vi "capex init.vi"(2 "GPIO registers":digitaldata={"transitions"=[], "data"=[[0, 0, 0, 0, 0, 0, 0, 0, 0, 0, 0, 0, 0, 0, 0, 0, 0, 0, 0, 0, 0, 0, 0, 0, 0, 0, 0, 0, 0, 0, 0, 0]]}) -> (0 "TC names default":string[](array[string]), 1 "DC defaults":dbl[](array[numeric]), 3 "AC defaults":dbl[](array[numeric]), 4 "Chiller defaults":dbl[](array[numeric]), 5 "AO names default":string[](array[string]), 6 "AI names default":string[](array[string]), 7 "Relay names default":string[](array[string]), 8 "AO defaults":dbl[](array[numeric]), 9 "Relay defaults":bool[](array[boolean]))   [LabVIEW 2013]
uses:
  <vilib>/Waveform/DTblOps.llb/DTbl Digital to Boolean Array.vi
  <resource>/objmgr/daqmx.rc
panel:
  in  "DC amps actual":dbl=60.0
  in  "DC volts actual":dbl=60.0
  in  "AC amps actual":dbl
  in  "AC volts actual":dbl
  in  "String 69":string="AI32"
  in  "String 68":string="AI31"
  in  "String 67":string="AI30"
  in  "String 66":string="AI29"
  in  "String 65":string="AI28"
  in  "String 64":string="AI27"
  in  "String 63":string="AI26"
  in  "String 62":string="AI25"
  in  "String 61":string="AI24"
  in  "String 60":string="AI23"
  in  "String 59":string="AI22"
  in  "String 58":string="AI21"
  in  "String 57":string="AI20"
  in  "String 56":string="AI19"
  in  "String 55":string="AI18"
  in  "String 54":string="AI17"
  in  "String 18":string="TC16"
  in  "String 17":string="TC15"
  out "hex integer string":string[](array[string])
  out "Array":tag[](array[tag])
  in  "Humidity process value":dbl
  in  "Temperature process value":dbl
  in  "Temperature setpoint":dbl
  in  "Humidity setpoint":dbl
  in  "String 53":string="Relay 4"
  in  "String 52":string="Relay 3"
  in  "String 51":string="Relay 2"
  in  "String 50":string="Relay 1"
  in  "String 49":string="AI16"
  in  "String 48":string="AI15"
  in  "String 47":string="AI14"
  in  "String 46":string="AI13"
  in  "String 45":string="AI12"
  in  "String 44":string="AI11"
  in  "String 43":string="AI10"
  in  "String 42":string="AI9"
  in  "String 41":string="AI8"
  in  "String 40":string="AI7"
  in  "String 39":string="AI6"
  in  "String 38":string="AI5"
  in  "String 37":string="AI4"
  in  "String 36":string="AI3"
  in  "String 35":string="AI2"
  in  "String 34":string="AI1"
  in  "Relay 4 default":bool
  in  "Relay 3 default":bool
  in  "Relay 2 default":bool
  in  "Relay 1 default":bool
  in  "Numeric 16":dbl
  in  "Numeric 15":dbl
  in  "Numeric 14":dbl
  in  "Numeric 13":dbl
  in  "Numeric 12":dbl
  in  "Numeric 11":dbl
  in  "Numeric 10":dbl
  in  "Numeric 9":dbl
  in  "Numeric 8":dbl
  in  "Numeric 7":dbl
  in  "Numeric 6":dbl
  in  "Numeric 5":dbl
  in  "Numeric 4":dbl
  in  "Numeric 3":dbl
  in  "Numeric 2":dbl
  in  "Numeric":dbl
  in  "String 33":string="AO16"
  in  "String 32":string="AO15"
  in  "String 31":string="AO14"
  in  "String 30":string="AO13"
  in  "String 29":string="AO12"
  in  "String 28":string="AO11"
  in  "String 27":string="AO10"
  in  "String 26":string="AO9"
  in  "String 25":string="AO8"
  in  "String 24":string="AO7"
  in  "String 23":string="AO6"
  in  "String 22":string="AO5"
  in  "String 21":string="AO4"
  in  "String 20":string="AO3"
  in  "String 19":string="AO2"
  in  "String 9":string="AO1"
  in  "Chiller pump default":dbl(ring) items=["Low", "Med", "High"]
  in  "Chiller temp default":dbl
  in  "DC OCP default":dbl
  in  "DC OVP default":dbl
  in  "DC amp default":dbl
  in  "DC volt default":dbl
  in  "AC frequency default":dbl=60.0
  in  "AC OCP default":dbl
  in  "AC OVP default":dbl
  in  "AC amp default":dbl
  in  "AC volt default":dbl
  in  "String 16":string="TC14"
  in  "String 15":string="TC13"
  in  "String 14":string="TC12"
  in  "String 13":string="TC11"
  in  "String 12":string="TC10"
  in  "String 11":string="TC9"
  in  "String 10":string="TC8"
  in  "String 8":string="TC7"
  in  "String 7":string="TC6"
  in  "String 6":string="TC5"
  in  "String 5":string="TC4"
  in  "String 4":string="TC3"
  in  "String 3":string="TC2"
  in  "String 2":string="TC1"
  # "Analog in"
  # "TC default names"
  # "Analog out"
  # "AC power starting values"
  # "DC power starting values"
  # "Chiller"
  # "Relays"
  # "Don't forget to set all items to default after editing!"
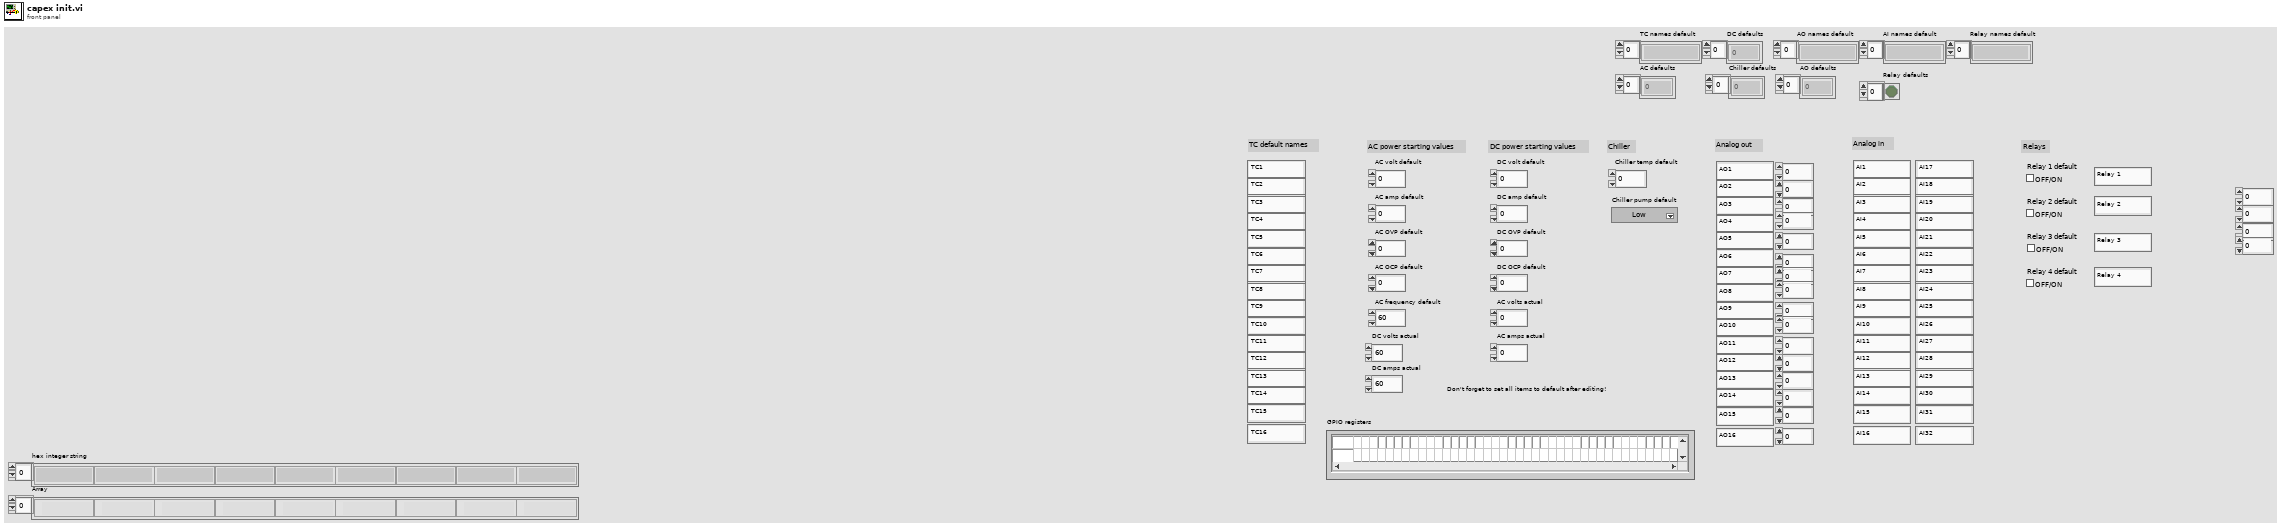
[diagram p1: front panel]
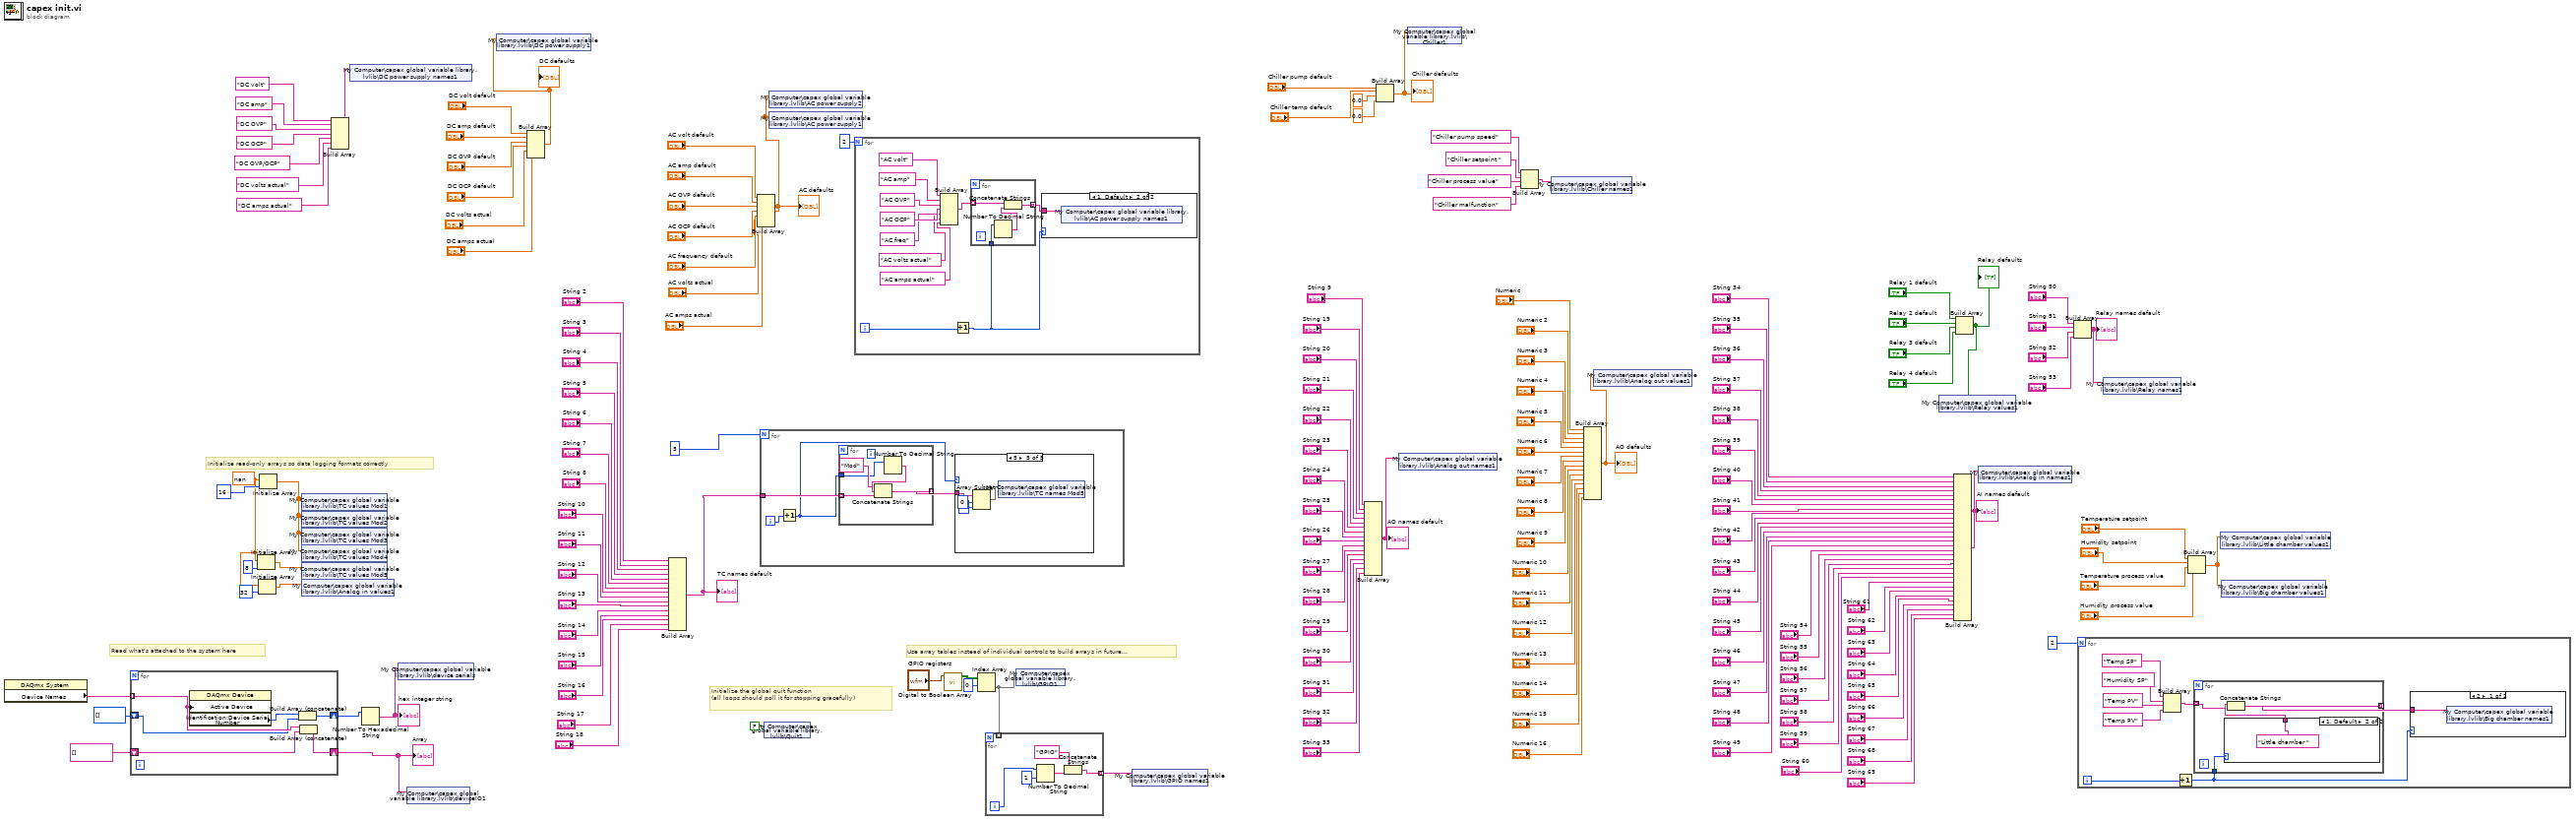
[diagram p0: block diagram]
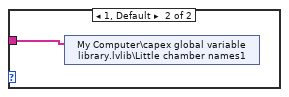
[diagram p2: hidden frame]
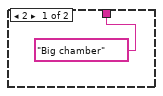
[diagram p3: hidden frame]
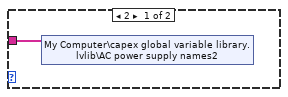
[diagram p4: hidden frame]
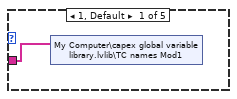
[diagram p5: hidden frame]
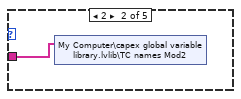
[diagram p6: hidden frame]
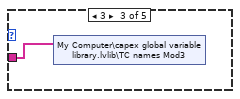
[diagram p7: hidden frame]
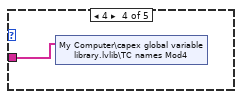
[diagram p8: hidden frame]
diagram:
  w27 = nan ("element")
  # "Initialize the global quit function\n(all loops should poll it for stopping gracefully)"
  # "Read what's attached to the system here"
  # "Initialize read-only arrays so data logging formats correctly"
  # "Use array tables instead of individual controls to build arrays in future..."
  n1 = property class="DAQmx System"() -> ("Device Names"=w36:tag[])  [unwired: 2 in, 2 out]
  n2 = for {
    tunnel: w36 -> [w159] mode=indexing
    shift-right: [w158] -> w32
    shift-left: tag[] [] -> [w160]
    shift-right: [w156] -> w34
    shift-left: u32[] [] -> [w155]
    n3 = property class="DAQmx Device"("Active Device"=w159) -> ("Identification:Device Serial Number"=w157:u32)  [unwired: 2 in, 2 out]
    n4 = Build Array (concatenate)(w157, w155) -> (w156:u32[])
    n5 = Build Array (concatenate)(w159, w160) -> (w158:tag[])
  }
  "Array" <- w32
  n6 = Initialize Array(w27, 8 ("dimension size")) -> (w29:dbl[])
  n7 = Initialize Array(w27, 32 ("dimension size")) -> (w28:dbl[])
  n8 = Initialize Array(w27, 16 ("dimension size")) -> (w37:dbl[])
  n9 = shared-variable "My Computer\\capex global variable library.lvlib\\TC values Mod1"(w37) -> ()  [unwired: 1 in, 1 out]
  n10 = shared-variable "My Computer\\capex global variable library.lvlib\\TC values Mod2"(w37) -> ()  [unwired: 1 in, 1 out]
  n11 = shared-variable "My Computer\\capex global variable library.lvlib\\TC values Mod3"(w37) -> ()  [unwired: 1 in, 1 out]
  n12 = shared-variable "My Computer\\capex global variable library.lvlib\\TC values Mod4"(w37) -> ()  [unwired: 1 in, 1 out]
  n13 = shared-variable "My Computer\\capex global variable library.lvlib\\TC values Mod5"(w29) -> ()  [unwired: 1 in, 1 out]
  n14 = shared-variable "My Computer\\capex global variable library.lvlib\\Analog in values1"(w28) -> ()  [unwired: 1 in, 1 out]
  n15 = Build Array("DC volt", "DC amp", "DC OVP", "DC OCP", "DC OVP/OCP", "DC volts actual", "DC amps actual") -> (w49:string[])
  n16 = shared-variable "My Computer\\capex global variable library.lvlib\\DC power supply names1"(w49) -> ()  [unwired: 1 in, 1 out]
  n17 = Number To Hexadecimal String(2:w34) -> (0:w31:string[])  [unwired: 1 in]
  "hex integer string" <- w31
  n18 = shared-variable "My Computer\\capex global variable library.lvlib\\device serials"(w31) -> ()  [unwired: 1 in, 1 out]
  n19 = shared-variable "My Computer\\capex global variable library.lvlib\\deviceIO1"(w32) -> ()  [unwired: 1 in, 1 out]
  n20 = Build Array("DC volt default", "DC amp default", "DC OVP default", "DC OCP default", "DC volts actual", "DC amps actual") -> (w70:dbl[])
  "DC defaults" <- w70
  n21 = shared-variable "My Computer\\capex global variable library.lvlib\\DC power supply1"(w70) -> ()  [unwired: 1 in, 1 out]
  n22 = Build Array("String 2", "String 3", "String 4", "String 5", "String 6", "String 7", "String 8", "String 10", "String 11", "String 12", "String 13", "String 14", "String 15", "String 16", "String 17", "String 18") -> (w73:string[])
  "TC names default" <- w73
  n23 = Build Array("AC volt default", "AC amp default", "AC OVP default", "AC OCP default", "AC frequency default", "AC volts actual", "AC amps actual") -> (w71:dbl[])
  "AC defaults" <- w71
  n24 = for {
    N: 5 -> [_]
    tunnel: w73 -> [w164]
    i -> [w162]
    n25 = Increment(x=w162) -> (x+1=w161:i32)
    n26 = for {
      tunnel: w164 -> [w177] mode=indexing
      tunnel: w161 -> [w174]
      tunnel: [w173] -> w163 mode=indexing
      n27 = Number To Decimal String(number=w174) -> (decimal integer string=w176:string)  [unwired: 1 in]
      n28 = Concatenate Strings("Mod" ("string"), w176, w177) -> (w173:string)
    }
    n29 = case shown="5" w161 {
      tunnel: w163 -> [w165 w166 w167 w168 w172]
      frame 1, Default {
        n30 = shared-variable "My Computer\\capex global variable library.lvlib\\TC names Mod1"(w165) -> ()  [unwired: 1 in, 1 out]
      }
      frame 2 {
        n31 = shared-variable "My Computer\\capex global variable library.lvlib\\TC names Mod2"(w166) -> ()  [unwired: 1 in, 1 out]
      }
      frame 3 {
        n32 = shared-variable "My Computer\\capex global variable library.lvlib\\TC names Mod3"(w167) -> ()  [unwired: 1 in, 1 out]
      }
      frame 4 {
        n33 = shared-variable "My Computer\\capex global variable library.lvlib\\TC names Mod4"(w168) -> ()  [unwired: 1 in, 1 out]
      }
      frame 5 {
        n34 = Array Subset(array=w172, index=0, length=8) -> (w169:string[])
        n35 = shared-variable "My Computer\\capex global variable library.lvlib\\TC names Mod5"(w169) -> ()  [unwired: 1 in, 1 out]
      }
    }
  }
  n36 = shared-variable "My Computer\\capex global variable library.lvlib\\Quit1"(FALSE ("Quit1")) -> ()  [unwired: 1 in, 1 out]
  n37 = shared-variable "My Computer\\capex global variable library.lvlib\\AC power supply2"(w71) -> ()  [unwired: 1 in, 1 out]
  n38 = shared-variable "My Computer\\capex global variable library.lvlib\\AC power supply1"(w71) -> ()  [unwired: 1 in, 1 out]
  n39 = for {
    N: 2 -> [_]
    i -> [w179]
    n40 = Build Array("AC volt", "AC amp", "AC OVP", "AC OCP", "AC freq", "AC volts actual", "AC amps actual") -> (w182:string[])
    n41 = Increment(x=w179) -> (x+1=w180:i32)
    n42 = for {
      tunnel: w182 -> [w194] mode=indexing
      tunnel: [w192] -> w181 mode=indexing
      tunnel: w180 -> [w191]
      n43 = Number To Decimal String(number=w191) -> (decimal integer string=w193:string)  [unwired: 1 in]
      n44 = Concatenate Strings(w194, w193) -> (w192:string)
    }
    n45 = case shown="1, Default" w180 {
      tunnel: w181 -> [w189 w190]
      frame 2 {
        n46 = shared-variable "My Computer\\capex global variable library.lvlib\\AC power supply names2"(w189) -> ()  [unwired: 1 in, 1 out]
      }
      frame 1, Default {
        n47 = shared-variable "My Computer\\capex global variable library.lvlib\\AC power supply names1"(w190) -> ()  [unwired: 1 in, 1 out]
      }
    }
  }
  n48 = call-poly <vilib>:"Digital to Boolean Array.vi"("digital data"="GPIO registers") -> ("boolean array"=w62:bool[][])  [unwired: 9 in, 1 out]
  n49 = Index Array(array=w62, index (row)=0) -> (element=w43:bool[])  [unwired: 1 in]
  n50 = for {
    tunnel: w43 -> [_] mode=indexing
    tunnel: [w195] -> w42 mode=indexing
    i -> [w196]
    n51 = Number To Decimal String(number=w196, width (-)=i16 1) -> (decimal integer string=w198:string)
    n52 = Concatenate Strings("GPIO" ("string"), w198) -> (w195:string)
  }
  n53 = shared-variable "My Computer\\capex global variable library.lvlib\\GPIO1"(w43) -> ()  [unwired: 1 in, 1 out]
  n54 = shared-variable "My Computer\\capex global variable library.lvlib\\GPIO names1"(w42) -> ()  [unwired: 1 in, 1 out]
  n55 = Build Array("String 9", "String 19", "String 20", "String 21", "String 22", "String 23", "String 24", "String 25", "String 26", "String 27", "String 28", "String 29", "String 30", "String 31", "String 32", "String 33") -> (w68:string[])
  "AO names default" <- w68
  n56 = Build Array("Chiller pump default", "Chiller temp default", 0.0 ("element"), 0.0 ("element")) -> (w69:dbl[])
  "Chiller defaults" <- w69
  n57 = shared-variable "My Computer\\capex global variable library.lvlib\\Analog out names1"(w68) -> ()  [unwired: 1 in, 1 out]
  n58 = shared-variable "My Computer\\capex global variable library.lvlib\\Chiller1"(w69) -> ()  [unwired: 1 in, 1 out]
  n59 = Build Array("Chiller pump speed", "Chiller setpoint ", "Chiller process value", "Chiller malfunction") -> (w44:string[])
  n60 = shared-variable "My Computer\\capex global variable library.lvlib\\Chiller names1"(w44) -> ()  [unwired: 1 in, 1 out]
  n61 = Build Array("Numeric", "Numeric 2", "Numeric 3", "Numeric 4", "Numeric 5", "Numeric 6", "Numeric 7", "Numeric 8", "Numeric 9", "Numeric 10", "Numeric 11", "Numeric 12", "Numeric 13", "Numeric 14", "Numeric 15", "Numeric 16") -> (w67:dbl[])
  "AO defaults" <- w67
  n62 = shared-variable "My Computer\\capex global variable library.lvlib\\Analog out values1"(w67) -> ()  [unwired: 1 in, 1 out]
  n63 = Build Array("String 34", "String 35", "String 36", "String 37", "String 38", "String 39", "String 40", "String 41", "String 42", "String 43", "String 44", "String 45", "String 46", "String 47", "String 48", "String 49", "String 54", "String 55", "String 56", "String 57", "String 58", "String 59", "String 60", "String 61", "String 62", "String 63", "String 64", "String 65", "String 66", "String 67", "String 68", "String 69") -> (w66:string[])
  "AI names default" <- w66
  n64 = Build Array("Relay 1 default", "Relay 2 default", "Relay 3 default", "Relay 4 default") -> (w65:bool[])
  "Relay defaults" <- w65
  n65 = shared-variable "My Computer\\capex global variable library.lvlib\\Relay values1"(w65) -> ()  [unwired: 1 in, 1 out]
  n66 = shared-variable "My Computer\\capex global variable library.lvlib\\Analog in names1"(w66) -> ()  [unwired: 1 in, 1 out]
  n67 = Build Array("String 50", "String 51", "String 52", "String 53") -> (w64:string[])
  "Relay names default" <- w64
  n68 = for {
    N: 2 -> [_]
    i -> [w201]
    n69 = Build Array("Temp SP", "Humidity SP", "Temp PV", "Temp PV") -> (w203:string[])
    n70 = Increment(x=w201) -> (x+1=w200:i32)
    n71 = for {
      tunnel: w203 -> [w210] mode=indexing
      tunnel: [w213] -> w202 mode=indexing
      tunnel: w200 -> [w212]
      n72 = case shown="1, Default" w212 {
        tunnel: ["Big chamber" "Little chamber "] -> w211
        frame 2 {
        }
        frame 1, Default {
        }
      }
      n73 = Concatenate Strings(w211, w210) -> (w213:string)
    }
    n74 = case shown="2" w200 {
      tunnel: w202 -> [w208 w209]
      frame 2 {
        n75 = shared-variable "My Computer\\capex global variable library.lvlib\\Big chamber names1"(w208) -> ()  [unwired: 1 in, 1 out]
      }
      frame 1, Default {
        n76 = shared-variable "My Computer\\capex global variable library.lvlib\\Little chamber names1"(w209) -> ()  [unwired: 1 in, 1 out]
      }
    }
  }
  n77 = shared-variable "My Computer\\capex global variable library.lvlib\\Relay names1"(w64) -> ()  [unwired: 1 in, 1 out]
  n78 = Build Array("Temperature setpoint", "Humidity setpoint", "Temperature process value", "Humidity process value") -> (w56:dbl[])
  n79 = shared-variable "My Computer\\capex global variable library.lvlib\\Little chamber values1"(w56) -> ()  [unwired: 1 in, 1 out]
  n80 = shared-variable "My Computer\\capex global variable library.lvlib\\Big chamber values1"(w56) -> ()  [unwired: 1 in, 1 out]
